vi "KH7008 Get All Channel Gains.vi"(8 "error in (no error)":errorcluster, 11 "Channel Params []":T1[](array[typedef])) -> (0 "error out":errorcluster, 3 "Gains []":dbl[](array[numeric]))   [LabVIEW 2019, in "Instrument.KH7008.lvclass"]
uses:
  Instrument.KH7008.lvclass
  typedefs/SetAll-Cluster.ctl
  typedefs/Channel-Enum.ctl
  typedefs/Gain-Enum.ctl
  typedefs/Filter-Enum.ctl
  typedefs/Shunt-Enum.ctl
  typedefs/Coupling-Enum.ctl
  typedefs/Input Configuration-Enum.ctl
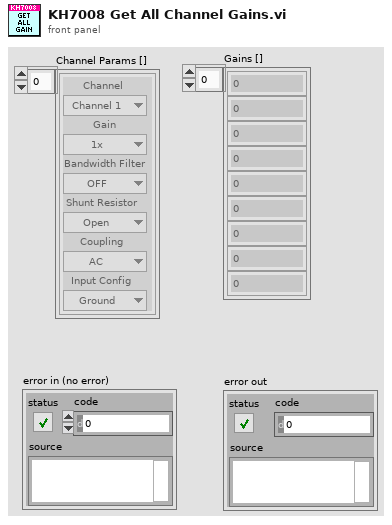
[diagram p1: front panel]
types:
  T1 = typedef "Instrument.KH7008.lvclass/SetAll-Cluster.ctl" = cluster{"Channel":T2, "Gain":T3, "Bandwidth Filter":T4, "Shunt Resistor":T5, "Coupling":T6, "Input Config":T7}
  T2 = typedef "Instrument.KH7008.lvclass/Channel-Enum.ctl" = enum16{"Channel 1", "Channel 2", "Channel 3", "Channel 4", "Channel 5", "Channel 6", "Channel 7", "Channel 8"}
  T3 = typedef "Instrument.KH7008.lvclass/Gain-Enum.ctl" = enum16{"1x", "10x", "100x", "1000x"}
  T4 = typedef "Instrument.KH7008.lvclass/Filter-Enum.ctl" = enum16{"OFF", "ON"}
  T5 = typedef "Instrument.KH7008.lvclass/Shunt-Enum.ctl" = enum16{"Open", "50 Ohms", "500 Ohms", "5k Ohms", "50k Ohms", "10M Ohm"}
  T6 = typedef "Instrument.KH7008.lvclass/Coupling-Enum.ctl" = enum16{"AC", "DC"}
  T7 = typedef "Instrument.KH7008.lvclass/Input Configuration-Enum.ctl" = enum16{"Ground", "SE+ (-gnd)", "SE- (+gnd)", "Differential"}
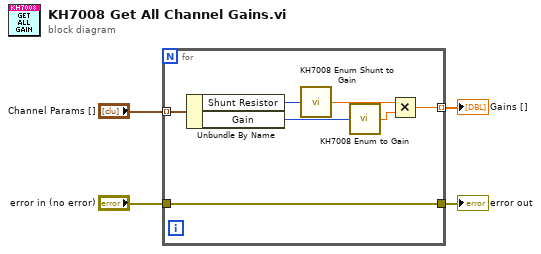
[diagram p0: block diagram]
diagram:
  n1 = for {
    tunnel: "Channel Params []" -> [w8] mode=indexing
    tunnel: [w11] -> w1 mode=indexing
    tunnel: "error in (no error)" -> [w5]
    tunnel: [w5] -> w3
    n2 = Unbundle By Name(w8) -> ("Shunt Resistor"=w7:T5, "Gain"=w6:T3)
    n3 = call "KH7008 Enum Shunt to Gain.vi"("Shunt Resistor"=w7) -> ("Gain (V/A)"=w10:dbl)
    n4 = call "KH7008 Enum to Gain.vi"("Gain"=w6) -> ("Gain (x)"=w9:dbl)
    n5 = Multiply(x=w10, y=w9) -> (x*y=w11:dbl)
  }
  "error out" <- w3
  "Gains []" <- w1
